vi "testTimestampInArray.vi"(8 "error in (no error)":errorcluster, 11 "TestCase in":refnum<class "EasyXMLTest.lvclass">) -> (0 "error out":errorcluster, 3 "TestCase out":refnum<class "EasyXMLTest.lvclass">)   [LabVIEW 2011, in "EasyXMLTest.lvclass"]
doc: "Verify that error in is not overwritten"
uses:
  EasyXMLTest.lvclass
panel:
  out "Generated XML String":string
  out "Produced Data":variant
  out "Input Data":variant
  out "XML String":string
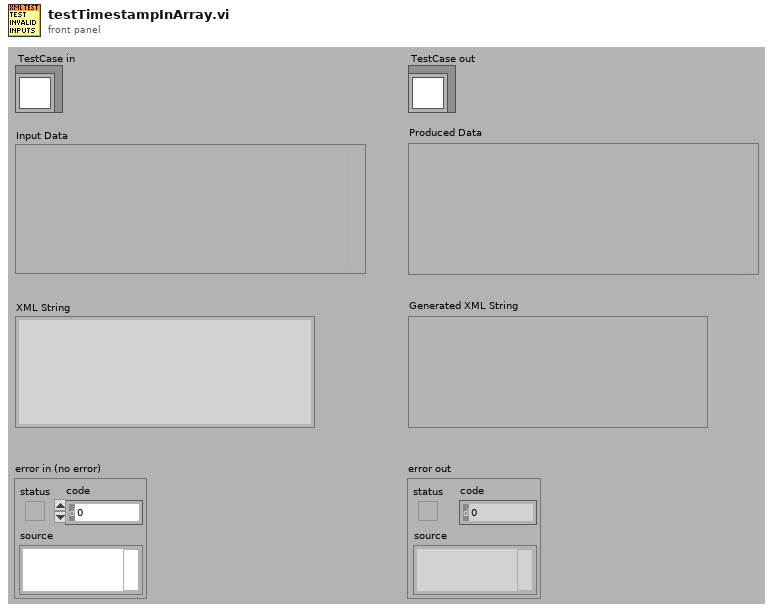
[diagram p1: front panel]
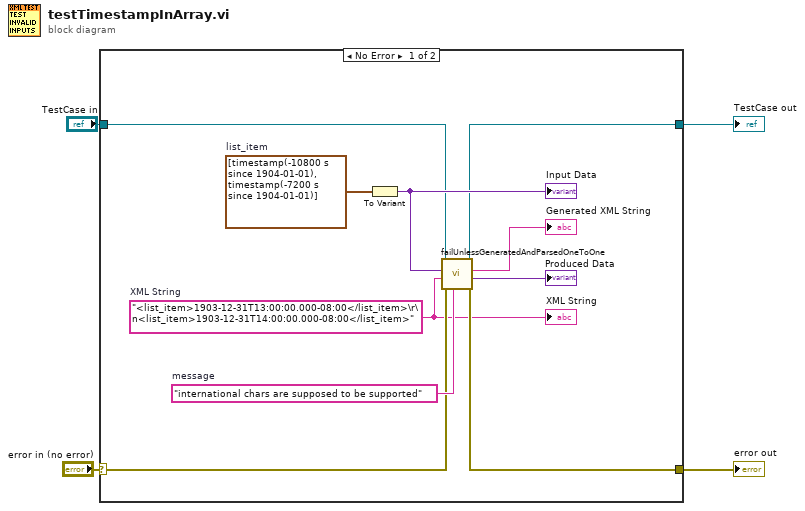
[diagram p0: block diagram]
diagram:
  n1 = case shown="No Error" "error in (no error)" {
    selector: "error in (no error)" -> [w11 w16]
    tunnel: [w10 w16] -> w2
    tunnel: [w6 w15] -> w1
    tunnel: "TestCase in" -> [w7 w15]
    frame No Error {
      w14 = timestamp[] [timestamp(-10800 s since 1904-01-01), timestamp(-7200 s since 1904-01-01)]  # list_item
      w12 = "international chars are supposed to be supported"  # message
      w8 = "<list_item>1903-12-31T13:00:00.000-08:00</list_item>\r\n<list_item>1903-12-31T14:00:00.000-08:00</list_item>"  # XML String
      n2 = To Variant(anything=w14) -> (Variant=w9:variant)
      "Input Data" <- w9
      n3 = call "failUnlessGeneratedAndParsedOneToOne.vi"("message (\"\")"=w12, "error in"=w11, "XML String"=w8, "Data"=w9, "EasyXMLTest in"=w7) -> ("error out"=w10:errorcluster, "Produced Data"=→"Produced Data":variant, "Generated XML String"=→"Generated XML String":string, "EasyXMLTest out"=w6:refnum<class "EasyXMLTest.lvclass">)  [unwired: 3 in]
      "XML String" <- w8
    }
    frame Error {
    }
  }
  "error out" <- w2
  "TestCase out" <- w1
